vi "IDNs.vi"(11 "uPluggable in":refnum<class "uPluggable.lvclass">) -> (2 "IDNs":string[](array[string]))   [LabVIEW 2023, in "uPlug.lvlib" / "uPluggable.lvclass"]
doc: "Use when multiple IDN strings are assigned to a single class.\n\nIf not overriden by the child, the default implementation by the abstract parent interface is to return the IDN method's output but in a single element array."
uses:
  uPluggable.lvclass
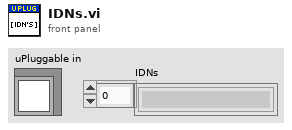
[diagram p1: front panel]
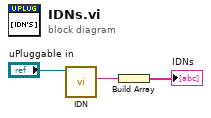
[diagram p0: block diagram]
diagram:
  n1 = call-dynamic "IDN.vi"("uPluggable in"="uPluggable in") -> ("IDN"=w2:string)  [unwired: 10 in]
  n2 = Build Array(w2) -> (→"IDNs":string[])
